vi "报警设置-回执解析.vi"(11 "完整输入":string="\u0001\u0003\u0004\u0014\u0000\u0000\u0000ÿÃ") -> (0 "有效数据？":bool, 2 "探头号":u16, 3 "限值":dbl)   [LabVIEW 2017]
uses:
  <vilib>/regexp/Match Regular Expression.xnode
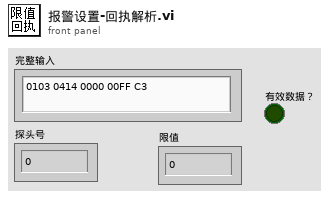
[diagram p1: front panel]
types:
  T1 = typedef "簇-输入.ctl" = cluster{"配置文件动作":T2, "数据输入":variant}
  T2 = typedef "枚举-配置文件动作.ctl" = enum16{"初始化加载配置", "读取配置", "写入-屏幕键盘", "写入-静音延迟", "写入-主要探头类型", "写入-串口配置", "写入-累积定时", "写入-导出定时", "保存配置到文件"}
  T3 = typedef "簇-配置文件内容.ctl" = cluster{"调试模式？":bool, "屏幕键盘？":bool, "软件版本":string, "静音延迟 s":u16, "主要探头类型":T4, "串口配置":cluster{"COM口":refnum<visa-resource-name>, "波特率":enum16{"9600", "19200"}, "读写超时ms":i16, "丢包判定次数":i16}, "定时配置-累积分段":T5, "定时配置-自动导出":cluster{"定时配置-自动导出":T5, "分别导出?":bool}}
  T4 = typedef "枚举-主要探头类型.ctl" = enum16{"网络探头", "串口探头"}
  T5 = typedef "簇-定时配置.ctl" = cluster{"定时模式":enum16{"绝对时间", "相对时间"}, "单位":enum16{"年", "月", "日", "时", "分"}, "间隔":u8, "目标时刻":timestamp}
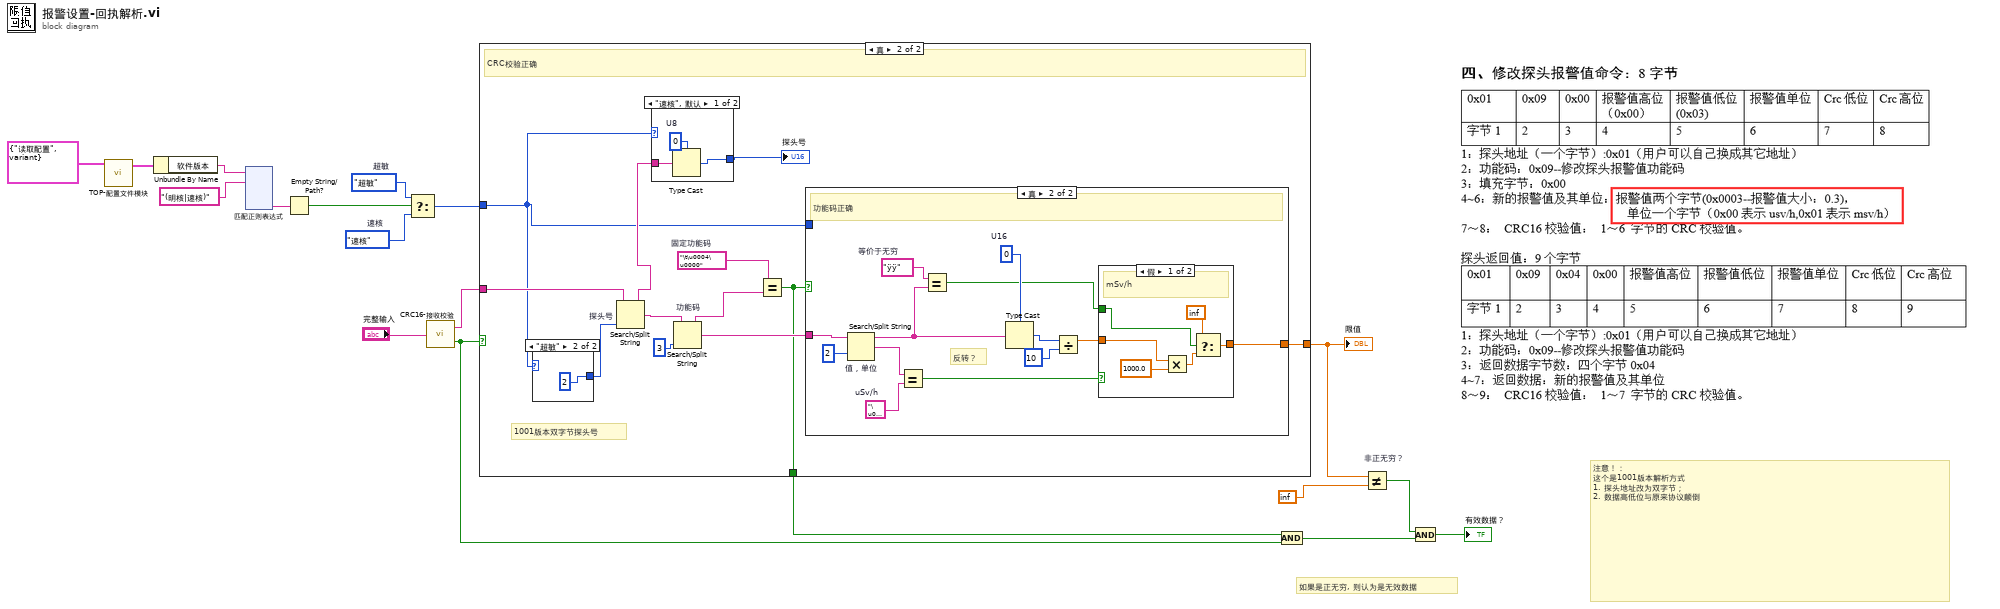
[diagram p0: block diagram]
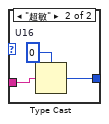
[diagram p3: hidden frame]
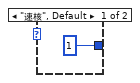
[diagram p4: hidden frame]
diagram:
  w3 = enum16{"速核", "超敏"}."速核"  # 速核
  w4 = enum16{"速核", "超敏"}."超敏"  # 超敏
  # "如果是正无穷, 则认为是无效数据"
  # "注意！：\n这个是1001版本解析方式\n1. 探头地址改为双字节；\n2. 数据高低位与原来协议颠倒"
  n1 = call "TOP-配置文件模块.vi"("输入"=T1 {"配置文件动作"=enum."读取配置", "数据输入"=variant}) -> ("配置文件"=w7:T3)  [unwired: 9 in, 1 out]
  n2 = Unbundle By Name(w7) -> ("软件版本"=w6:string)
  n3 = xnode "匹配正则表达式"("输入字符串"=w6, "正则表达式"="(明核|速核)") -> ("子匹配 1"=w5:string)  [unwired: 4 in, 5 out]
  n4 = Empty String/Path?(string/path=w5) -> (empty?=w1:bool)
  n5 = Select(t=w4, s=w1, f=w3) -> (s? t:f=w2:enum16{"速核", "超敏"})
  n6 = call "CRC16-接收校验.vi"("读取缓冲区"="完整输入") -> ("净数据"=w17:string, "CRC？"=w16:bool)
  n7 = case shown="真" w16 {
    tunnel: w17 -> [_ w25]
    tunnel: [_ w28] -> w12
    tunnel: [_ w23] -> w15
    tunnel: w2 -> [_ w19]
    frame False {
    }
    frame True {
      w26 = "\t\u0004\u0000"  # 固定功能码
      # "1001版本双字节探头号"
      # "CRC校验正确"
      n8 = case shown="\"超敏\"" w19 {
        tunnel: [1 ("偏移量(0)") 2 ("偏移量(0)")] -> w22
        frame "速核", Default {
        }
        frame "超敏" {
        }
      }
      n9 = Search/Split String "探头号"(string=w25, offset (0)=w22) -> (substring before match=w21:string, match + rest of string=w24:string)  [unwired: 1 in, 1 out]
      n10 = case shown="\"速核\", 默认" w19 {
        tunnel: w21 -> [w31 w36]
        tunnel: [w32 w34] -> w20
        frame "速核", Default {
          w33 = u8 0  # U8
          n11 = Type Cast(type=w33, x=w31) -> (*(type *) &x=w32:u8)
        }
        frame "超敏" {
          w35 = u16 0  # U16
          n12 = Type Cast(type=w35, x=w36) -> (*(type *) &x=w34:u16)
        }
      }
      "探头号" <- w20
      n13 = Search/Split String "功能码"(string=w24, offset (0)=3 ("偏移量(0)")) -> (substring before match=w27:string, match + rest of string=w29:string)  [unwired: 1 in, 1 out]
      n14 = Equal?(x=w26, y=w27) -> (x = y?=w23:bool)
      n15 = case shown="真" w23 {
        tunnel: w29 -> [_ w51]
        tunnel: [_ w45] -> w28
        tunnel: w19 -> [_ _]
        frame False {
          # "功能码错误"
        }
        frame True {
          w41 = "ÿÿ"  # 等价于无穷
          w47 = "\u0000"  # uSv/h
          w49 = u16 0  # U16
          # "反转？"
          # "功能码正确"
          n16 = Search/Split String "值，单位"(string=w51, offset (0)=2 ("偏移量(0)")) -> (substring before match=w39:string, match + rest of string=w48:string)  [unwired: 1 in, 1 out]
          n17 = Equal?(x=w48, y=w47) -> (x = y?=w46:bool)
          n18 = Equal?(x=w41, y=w39) -> (x = y?=w40:bool)
          n19 = Type Cast(type=w49, x=w39) -> (*(type *) &x=w44:u16)
          n20 = Divide(x=w44, y=u16 10) -> (x/y=w43:dbl)
          n21 = case shown="假" w46 {
            tunnel: w43 -> [w57 w58]
            tunnel: [w52 w58] -> w45
            tunnel: w40 -> [w55 _]
            frame False {
              # "mSv/h"
              n22 = Multiply(x=w57, y=1000.0) -> (x*y=w53:dbl)
              n23 = Select(t=inf, s=w55, f=w53) -> (s? t:f=w52:dbl)
            }
            frame True {
              # "uSv/h"
            }
          }
        }
      }
    }
  }
  "限值" <- w12
  n24 = And(x=w15, y=w16) -> (x .and. y?=w14:bool)
  n25 = Not Equal? "非正无穷？"(x=w12, y=inf) -> (x != y?=w10:bool)
  n26 = And(x=w10, y=w14) -> (x .and. y?=→"有效数据？":bool)
